vi "Read channel active (index).vi"(8 "error in (no error)":errorcluster, 11 "OSA300 in":refnum<class "OSA300.lvclass">) -> (0 "error out":errorcluster, 2 "channel active (index)":i32, 3 "OSA300 out":refnum<class "OSA300.lvclass">)   [LabVIEW 2010, in "OSA300.lvclass"]
uses:
  OSA300.lvclass
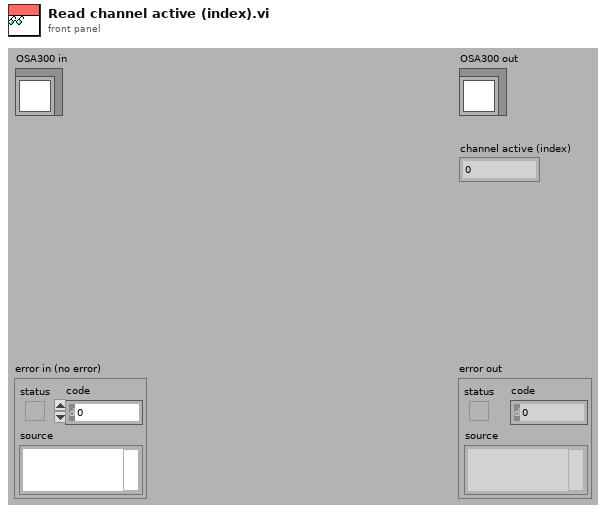
[diagram p1: front panel]
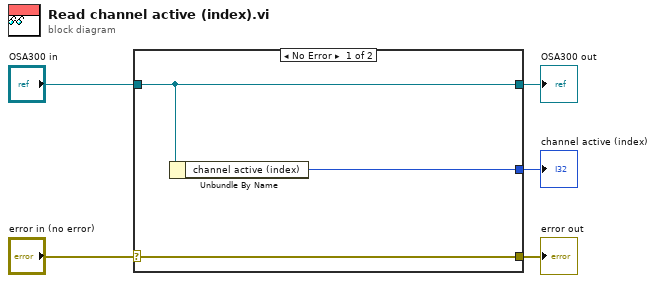
[diagram p0: block diagram]
diagram:
  n1 = case shown="No Error" "error in (no error)" {
    selector: "error in (no error)" -> [w8 w9]
    tunnel: [w8 w9] -> w4
    tunnel: [w7 w10] -> w2
    tunnel: "OSA300 in" -> [w7 w10]
    tunnel: [w6 _] -> w1
    frame No Error {
      n2 = Unbundle By Name(w7) -> ("channel active (index)"=w6:i32)
    }
    frame Error {
    }
  }
  "error out" <- w4
  "OSA300 out" <- w2
  "channel active (index)" <- w1
